vi "suscriptor.vi"() -> ()   [LabVIEW 2020]
uses:
  <vilib>/LabVIEW Open Source Project/MQTT Client/Client class/Client.lvclass/Client.ctl
  <vilib>/LabVIEW Open Source Project/MQTT Connection/MQTT_Base/Base Class/MQTT_Base.lvclass/MQTT_Base.ctl
  <vilib>/LabVIEW Open Source Project/MQTT TCP Connection/MQTT_TCP/Connection/TCPConnection.lvclass
  C:/Program Files (x86)/National Instruments/LabVIEW 2020/vi.lib/LabVIEW Open Source Project/Connection/Connection/Connection.lvclass
  <vilib>/LabVIEW Open Source Project/MQTT Client/Client class/Client.lvclass
  C:/Program Files (x86)/National Instruments/LabVIEW 2020/vi.lib/LabVIEW Open Source Project/MQTT Connection/MQTT_Base/Base Class/MQTT_Base.lvclass
  <vilib>/LabVIEW Open Source Project/MQTT Control Packets/Control Packets/PUBLISH/PUBLISH.lvclass
  <vilib>/LabVIEW Open Source Project/MQTT Connection/MQTT_Base/Base Class/MQTT_Base.lvclass
  <vilib>/LabVIEW Open Source Project/Connection/Connection.LocalQueue/Connection.LocalQueue.lvclass
  <vilib>/LabVIEW Open Source Project/Connection/Connection/Connection.lvclass
panel:
  out "Waveform Chart":dbl(graph)
  in  "Thermometer":dbl(slide) scale=0.0..100.0
  out "Unsuback":bool
  out "Suback":bool
  in  "Subscribe":bool
  in  "Connection":bool
  in  "Stop Client":bool
  out "last error":errorcluster
types:
  T1 = typedef "MQTT Client.lvlib/Client.lvclass/Public Events -- cluster.ctl" = cluster{"Connection Status":refnum<user-event>, "Connected":refnum<user-event>, "Application Message":refnum<user-event>}
  T2 = typedef "MQTT Base.lvlib/MQTT_Base.lvclass/Public Events -- cluster.ctl" = cluster{"Stop Event":refnum<user-event>, "Error Event":refnum<user-event>, "Inbound Message":refnum<user-event>}
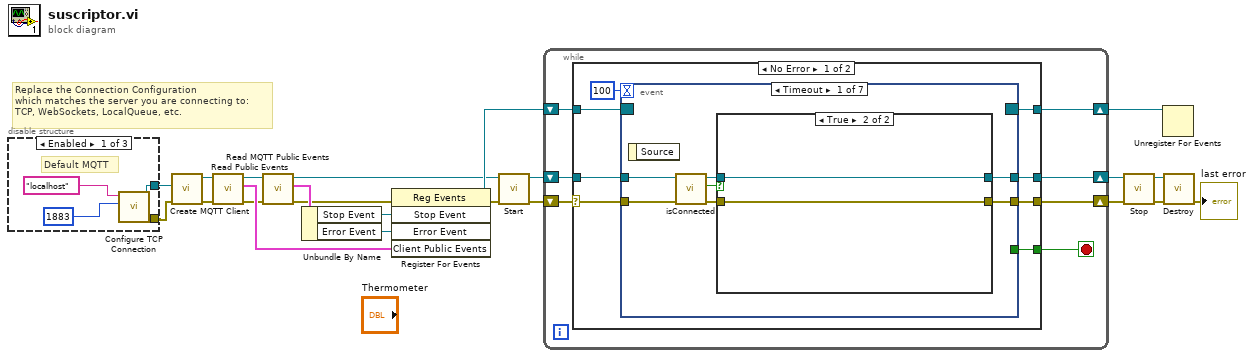
[diagram p0: block diagram]
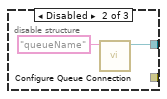
[diagram p2: hidden frame]
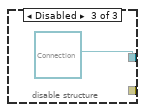
[diagram p3: hidden frame]
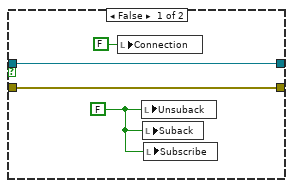
[diagram p4: hidden frame]
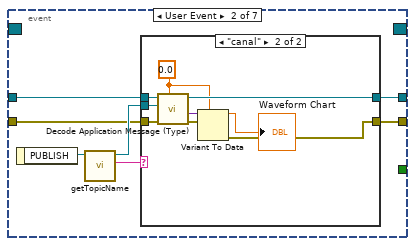
[diagram p5: hidden frame]
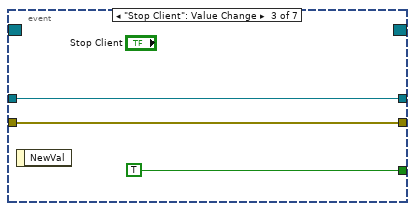
[diagram p7: hidden frame]
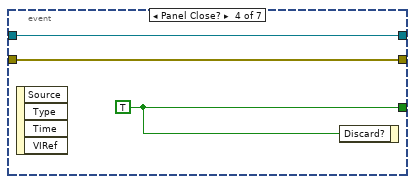
[diagram p8: hidden frame]
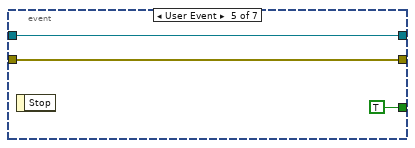
[diagram p9: hidden frame]
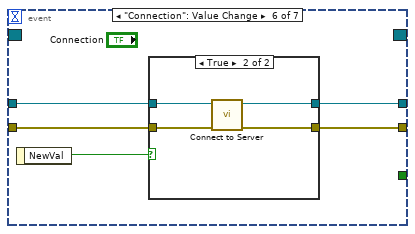
[diagram p10: hidden frame]
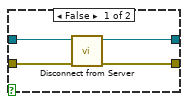
[diagram p11: hidden frame]
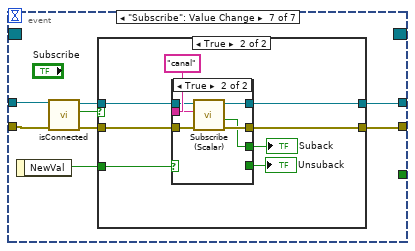
[diagram p12: hidden frame]
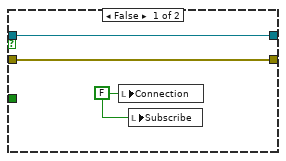
[diagram p13: hidden frame]
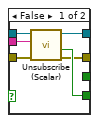
[diagram p14: hidden frame]
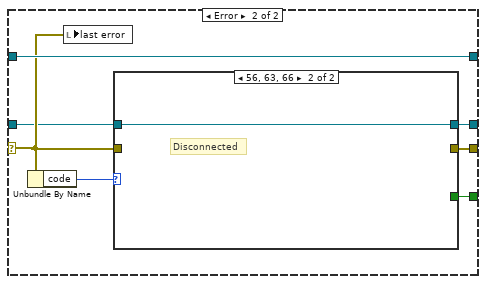
[diagram p15: hidden frame]
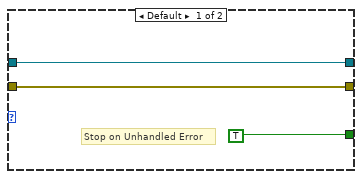
[diagram p16: hidden frame]
diagram:
  # "Replace the Connection Configuration\nwhich matches the server you are connecting to:\nTCP, WebSockets, LocalQueue, etc."
  n1 = disable-structure shown="Enabled" {
    disable-tunnel: [w24 w28 refnum<class "Connection.lvclass"> refnum ("Connection Configuration")] -> w22
    disable-tunnel: [w23 _ _] -> w1
    frame Enabled {
      # "Default MQTT"
      n2 = call <vilib>:"Configure TCP Connection.vi"("remote port (80)"=u16 1883, "address (localhost)"="localhost") -> ("error out"=w23:errorcluster, "TCPConnection"=w24:refnum<class "TCPConnection.lvclass">)  [unwired: 8 in]
    }
    frame Disabled {
      n3 = call <vilib>:"Configure Queue Connection.vi"("Queue Name"="queueName") -> ("Connection.LocalQueue"=w28:refnum<class "Connection.LocalQueue.lvclass">)  [unwired: 9 in, 1 out]
    }
    frame Disabled {
    }
  }
  n4 = call <vilib>:"Create MQTT Client.vi"("error in (no error)"=w1, "Connection Configuration"=w22) -> ("error out"=w4:errorcluster, "Client out"=w2:refnum<class "Client.lvclass">)  [unwired: 8 in]
  n5 = call <vilib>:"Read Public Events.vi"("error in (no error)"=w4, "Client in"=w2) -> ("error out"=w5:errorcluster, "Client Public Events"=w7:T1, "Client out"=w3:refnum<class "Client.lvclass">)  [unwired: 7 in]
  n6 = call <vilib>:"Read MQTT Public Events.vi"("error in (no error)"=w5, "MQTT_Base in"=w3) -> ("error out"=w6:errorcluster, "MQTT Public Events"=w14:T2, "MQTT_Base out"=w9:refnum<class "Client.lvclass">)  [unwired: 7 in]
  n7 = Unbundle By Name(w14) -> ("Stop Event"=w12:refnum<user-event>, "Error Event"=w13:refnum<user-event>)
  n8 = register-events(error in=w6, w12, w13, w7) -> (reference out=w10:refnum<event-registration>, error out=w8:errorcluster)  [unwired: 1 in]
  n9 = call <vilib>:"Start.vi"("error in (no error)"=w8, "MQTT_Base in"=w9) -> ("error out"=w20:errorcluster, "MQTT_Base out"=w19:refnum<class "Client.lvclass">)  [unwired: 7 in, 1 out]
  n10 = while {
    shift-right: [w35] -> w11
    shift-left: w10 -> [w36]
    shift-right: [w32] -> w16
    shift-left: w19 -> [w33]
    shift-right: [w34] -> w18
    shift-left: w20 -> [w30]
    stop <- w31 stop-if-true
    n11 = case shown="No Error" w30 {
      selector: w30 -> [w37 w132]
      tunnel: w36 -> [w44 w135]
      tunnel: [w43 w135] -> w35
      tunnel: [w42 w130] -> w34
      tunnel: w33 -> [w40 w131]
      tunnel: [w39 w134] -> w32
      tunnel: [w38 w129] -> w31
      frame No Error {
        n12 = event shown="[0] Timeout" {
          selector: w44 -> [_ _ _ _ _ _ _]
          dyn-events: [_ _ _ _ _ _ _] -> w43
          timeout: 100 -> [_ _ _ _ _ _ _]
          tunnel: w37 -> [w47 w61 w77 w79 w84 w85 w103]
          tunnel: [w50 w58 w77 w79 w84 w86 w104] -> w42
          tunnel: [_ _ TRUE w81 TRUE _ _] -> w38
          tunnel: w40 -> [w49 w62 w78 w80 w82 w89 w102]
          tunnel: [w51 w60 w78 w80 w82 w87 w105] -> w39
          event Timeout {
            n13 = event-data() -> ()  [unwired: 1 in, 1 out]
            n14 = call <vilib>:"isConnected.vi"("error in (no error)"=w47, "Client in"=w49) -> ("error out"=w46:errorcluster, "connected"=w45:bool, "Client out"=w48:refnum<class "Client.lvclass">)  [unwired: 7 in]
            n15 = case shown="True" w45 {
              tunnel: [w55 w57] -> w51
              tunnel: [w54 w56] -> w50
              tunnel: w48 -> [w55 w57]
              tunnel: w46 -> [w54 w56]
              frame False {
                w53 = FALSE
                n16 = local write "Connection"(FALSE ("Connection")) -> ()
                n17 = local write "Unsuback"(w53) -> ()
                n18 = local write "Suback"(w53) -> ()
                n19 = local write "Subscribe"(w53) -> ()
              }
              frame True {
              }
            }
          }
          event User Event {
            n20 = event-data() -> ("PUBLISH"=w64:refnum<class "PUBLISH.lvclass">)  [unwired: 1 in]
            n21 = call <vilib>:"getTopicName.vi"("PUBLISH in"=w64) -> ("Topic"=w59:string, "PUBLISH out"=w63:refnum<class "PUBLISH.lvclass">)  [unwired: 8 in, 1 out]
            n22 = case shown="\"canal\"" w59 {
              tunnel: w63 -> [_ w68]
              tunnel: w62 -> [w66 w74]
              tunnel: w61 -> [w65 w72]
              tunnel: [w66 w73] -> w60
              tunnel: [w65 w75] -> w58
              frame Default {
              }
              frame "canal" {
                w70 = 0.0
                n23 = call <vilib>:"Decode Application Message (Type).vi"("Type"=w70, "error in (no error)"=w72, "PUBLISH"=w68, "Client in"=w74) -> ("error out"=w71:errorcluster, "Payload"=w69:variant, "Client out"=w73:refnum<class "Client.lvclass">)  [unwired: 4 in, 1 out]
                n24 = Variant To Data(error in=w71, type=w70, Variant=w69) -> (data=→"Waveform Chart":dbl, error out=w75:errorcluster)
              }
            }
          }
          event "Stop Client": Value Change {
            n25 = event-data() -> ()  [unwired: 1 in, 1 out]
          }
          event Panel Close? {
            w81 = TRUE
            n26 = event-data() -> ()  [unwired: 1 in, 4 out]
            n27 = event-data("Discard?"=w81) -> ()  [unwired: 1 in, 1 out]
          }
          event User Event {
            n28 = event-data() -> ()  [unwired: 1 in, 1 out]
          }
          event "Connection": Value Change {
            n29 = event-data() -> ("NewVal"=w88:bool)  [unwired: 1 in]
            n30 = case shown="True" w88 {
              tunnel: w89 -> [w93 w97]
              tunnel: [w92 w94] -> w87
              tunnel: [w91 w95] -> w86
              tunnel: w85 -> [w90 w96]
              frame False {
                n31 = call <vilib>:"Disconnect from Server.vi"("error in (no error)"=w90, "Client in"=w93) -> ("error out"=w91:errorcluster, "Client out"=w92:refnum<class "Client.lvclass">)  [unwired: 7 in, 1 out]
              }
              frame True {
                n32 = call <vilib>:"Connect to Server.vi"("error in (no error)"=w96, "Client in"=w97) -> ("error out"=w95:errorcluster, "Client out"=w94:refnum<class "Client.lvclass">)  [unwired: 6 in, 2 out]
              }
            }
          }
          event "Subscribe": Value Change {
            n33 = event-data() -> ("NewVal"=w98:bool)  [unwired: 1 in]
            n34 = call <vilib>:"isConnected.vi"("error in (no error)"=w103, "Client in"=w102) -> ("error out"=w100:errorcluster, "connected"=w99:bool, "Client out"=w101:refnum<class "Client.lvclass">)  [unwired: 7 in]
            n35 = case shown="True" w99 {
              tunnel: [w108 w116] -> w105
              tunnel: [w107 w115] -> w104
              tunnel: w101 -> [w108 w114]
              tunnel: w100 -> [w107 w113]
              tunnel: w98 -> [_ w111]
              frame False {
                w106 = FALSE ("Connection")
                n36 = local write "Connection"(w106) -> ()
                n37 = local write "Subscribe"(w106) -> ()
              }
              frame True {
                n38 = case shown="True" w111 {
                  tunnel: [w117 w125] -> w116
                  tunnel: [w118 w124] -> w115
                  tunnel: w114 -> [w122 w128]
                  tunnel: w113 -> [w121 w127]
                  tunnel: "canal" ("Topic Name (empty: Payload name)") -> [w120 w126]
                  tunnel: [_ w123] -> w110
                  tunnel: [w119 _] -> w109
                  frame False {
                    n39 = call <vilib>:"Unsubscribe (Scalar).vi"("error in (no error)"=w121, "Topic Filter"=w120, "Client in"=w122) -> ("error out"=w118:errorcluster, "Ack"=w119:bool, "Client out"=w117:refnum<class "Client.lvclass">)  [unwired: 6 in]
                  }
                  frame True {
                    n40 = call <vilib>:"Subscribe (Scalar).vi"("error in (no error)"=w127, "Topic Filter"=w126, "Client in"=w128) -> ("error out"=w124:errorcluster, "Ack"=w123:bool, "Client out"=w125:refnum<class "Client.lvclass">)  [unwired: 6 in]
                  }
                }
                "Unsuback" <- w109
                "Suback" <- w110
              }
            }
          }
        }
      }
      frame Error {
        n41 = Unbundle By Name(w132) -> ("code"=w133:i32)
        n42 = local write "last error"(w132) -> ()
        n43 = case shown="56, 63, 66" w133 {
          tunnel: w131 -> [w138 w139]
          tunnel: [w138 w139] -> w134
          tunnel: w132 -> [w137 _]
          tunnel: [w137 _] -> w130
          tunnel: [TRUE _] -> w129
          frame Default {
            # "Stop on Unhandled Error"
          }
          frame 56, 63, 66 {
            # "Disconnected"
          }
        }
      }
    }
  }
  n44 = call <vilib>:"Stop.vi"("error in (no error)"=w18, "MQTT_Base in"=w16) -> ("error out"=w17:errorcluster, "MQTT_Base out"=w15:refnum<class "Client.lvclass">)  [unwired: 7 in, 1 out]
  n45 = Unregister For Events(event registration refnum=w11) -> ()  [unwired: 1 in, 1 out]
  n46 = call <vilib>:"Destroy.vi"("error in (no error)"=w17, "MQTT_Base in"=w15) -> ("error out"=→"last error":errorcluster)  [unwired: 8 in, 1 out]
